vi "VI Snippets.vi"(6 "args":string[](array[string]), 7 "QD Plugins Dir":path, 8 "error in (no error)":errorcluster, 9 "Shift?":bool, 10 "Focus":enum8{"FP", "BD"}(ring), 11 "VI Refnum":refnum<vi>) -> (0 "error out":errorcluster)   [LabVIEW 2018]
doc: "Imports or exports a VI Snippet (*.png) image programmatically. Import opens a preview dialog to select a VI Snippet (*.png) from the <b>QuickDrop\\plugins\\Snippets</b> directory. Export prompts the user where to save the VI Snippet (*.png). On export, if nothing is selected the entire VI is exported. Otherwise only the selected Block Diagram GObjects are exported.\n\n[SCRIPT]\nimport=Import VI Snippet\nexport=Export VI Snippet"
uses:
  VI Snippets.llb/VI Snippets.lvlib
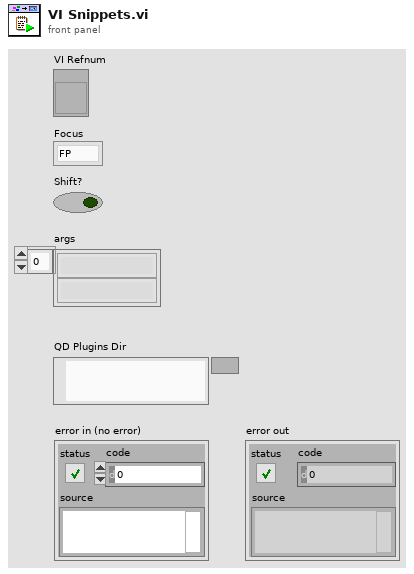
[diagram p1: front panel]
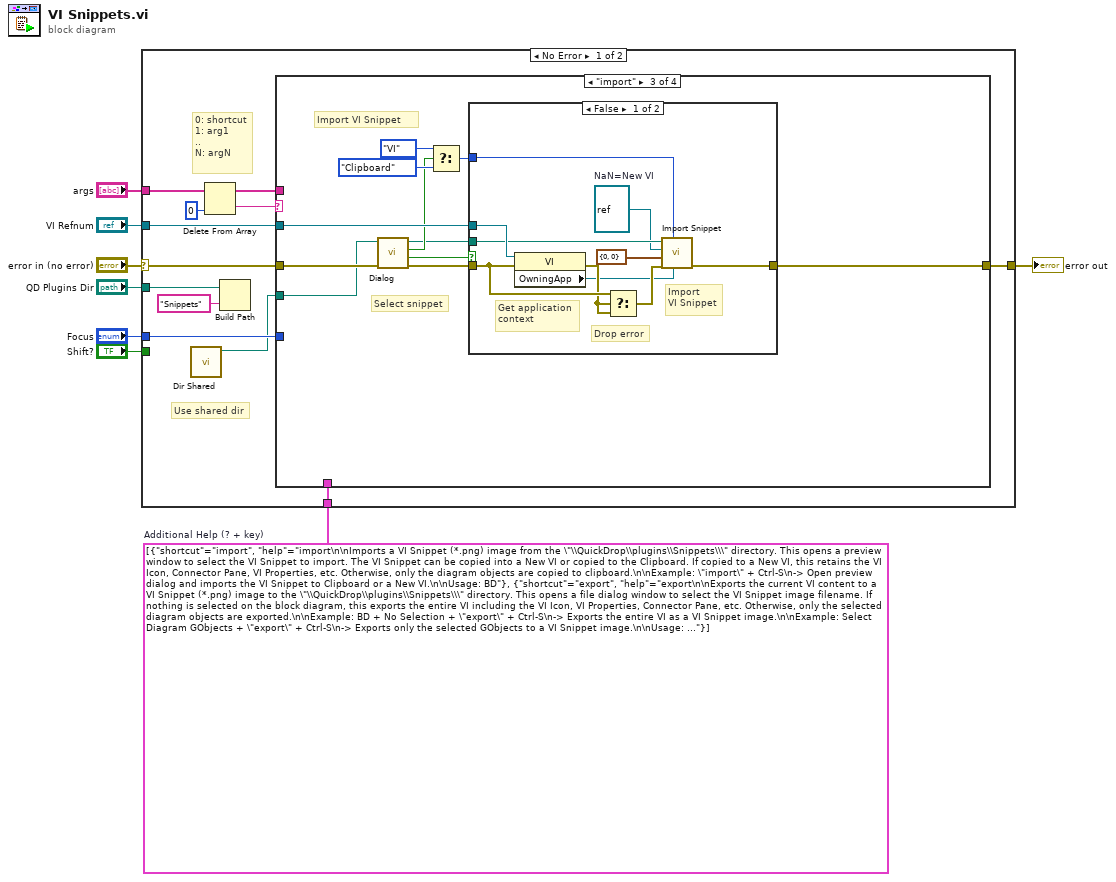
[diagram p0: block diagram]
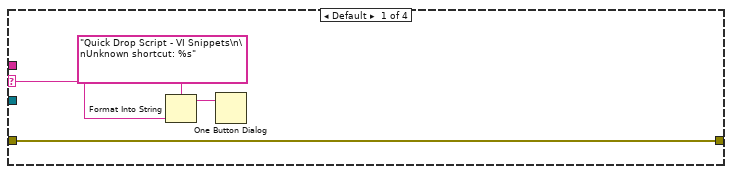
[diagram p2: hidden frame]
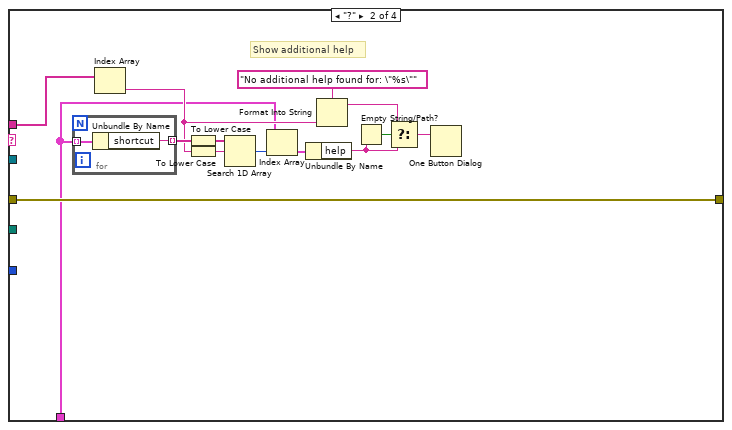
[diagram p3: hidden frame]
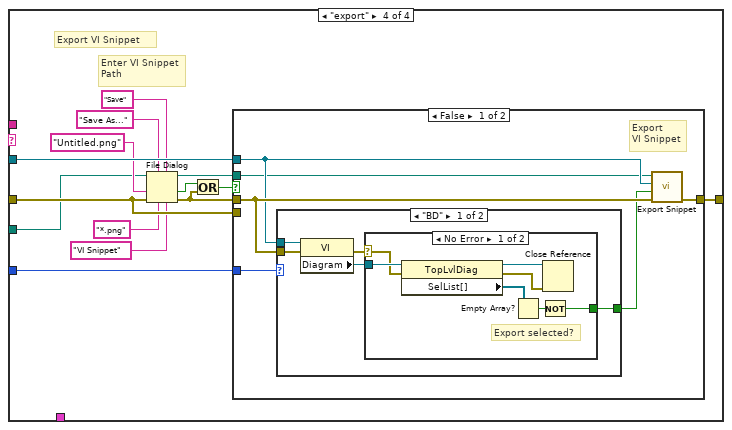
[diagram p5: hidden frame]
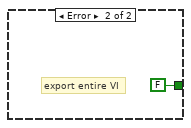
[diagram p6: hidden frame]
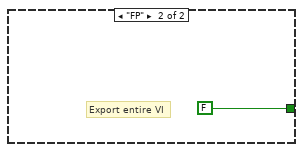
[diagram p7: hidden frame]
diagram:
  w1 = cluster{"shortcut":string, "help":string}[] [{"shortcut"="import", "help"="import\n\nImports a VI Snippet (*.png) image from the \"\\QuickDrop\\plugins\\Snippets\\\" directory. This opens a preview window to select the VI Snippet to import. The VI Snippet can be copied into a New VI or copied to the Clipboard. If copied to a New VI, this retains the VI Icon, Connector Pane, VI Properties, etc. Otherwise, only the diagram objects are copied to clipboard.\n\nExample: \"import\" + Ctrl-S\n-> Open preview dialog and imports the VI Snippet to Clipboard or a New VI.\n\nUsage: BD"}, {"shortcut"="export", "help"="export\n\nExports the current VI content to a VI Snippet (*.png) image to the \"\\QuickDrop\\plugins\\Snippets\\\" directory. This opens a file dialog window to select the VI Snippet image filename. If nothing is selected on the block diagram, this exports the entire VI including the VI Icon, VI Properties, Connector Pane, etc. Otherwise, only the selected diagram objects are exported.\n\nExample: BD + No Selection + \"export\" + Ctrl-S\n-> Exports the entire VI as a VI Snippet image.\n\nExample: Select Diagram GObjects + \"export\" + Ctrl-S\n-> Exports only the selected GObjects to a VI Snippet image.\n\nUsage: BD\n"}]  # Additional Help (? + key)
  n1 = case shown="No Error" "error in (no error)" {
    selector: "error in (no error)" -> [w16 w98]
    tunnel: "VI Refnum" -> [w12 _]
    tunnel: "Focus" -> [w11 _]
    tunnel: "Shift?" -> [_ _]
    tunnel: "args" -> [w19 _]
    tunnel: [w15 w98] -> w3
    tunnel: "QD Plugins Dir" -> [w14 _]
    tunnel: w1 -> [w10 _]
    frame No Error {
      # "Use shared dir"
      # "0: shortcut\n1: arg1\n..\nN: argN"
      n2 = call "Dir Shared.vi"() -> ("Shared Dir"=w9:path)  [unwired: 11 in]
      n3 = Delete From Array(array=w19, index=0) -> (deleted portion=w18:string, array with subset deleted=w17:string[])  [unwired: 1 in]
      n4 = Build Path(base path=w14, name or relative path="Snippets") -> ()  [unwired: 1 out]
      n5 = case shown="\"import\"" w18 {
        selector: w18 -> [w21 _ _ _]
        tunnel: [w24 w26 w51 w75] -> w15
        tunnel: w16 -> [w24 w26 w46 w72]
        tunnel: w17 -> [_ w27 _ _]
        tunnel: w9 -> [_ _ w42 w70]
        tunnel: w12 -> [_ _ w50 w74]
        tunnel: w11 -> [_ _ _ w73]
        tunnel: w10 -> [_ w25 _ _]
        frame Default {
          n6 = Format Into String(format string="Quick Drop Script - VI Snippets\n\nUnknown shortcut: %s", w21) -> (resulting string=w22:string)  [unwired: 2 in, 1 out]
          n7 = One Button Dialog(message=w22) -> ()  [unwired: 1 in, 1 out]
        }
        frame "?" {
          # "Show additional help"
          n8 = for {
            tunnel: w25 -> [w40] mode=indexing
            tunnel: [w39] -> w38 mode=indexing
            n9 = Unbundle By Name(w40) -> ("shortcut"=w39:string)
          }
          n10 = Index Array(array=w27) -> (element=w30:string)  [unwired: 1 in]
          n11 = To Lower Case(string=w38) -> (all lower case string=w37:string[])
          n12 = To Lower Case(string=w30) -> (all lower case string=w36:string)
          n13 = Search 1D Array(1D array=w37, element=w36) -> (index of element=w35:i32)  [unwired: 1 in]
          n14 = Index Array(array=w25, index=w35) -> (element=w34:cluster{"shortcut":string, "help":string})
          n15 = Unbundle By Name(w34) -> ("help"=w32:string)
          n16 = Format Into String(format string="No additional help found for: \"%s\"", w30) -> (resulting string=w29:string)  [unwired: 2 in, 1 out]
          n17 = Empty String/Path?(string/path=w32) -> (empty?=w33:bool)
          n18 = Select(t=w29, s=w33, f=w32) -> (s? t:f=w31:string)
          n19 = One Button Dialog(message=w31) -> ()  [unwired: 1 in, 1 out]
        }
        frame "import" {
          # "Import VI Snippet"
          # "Select snippet"
          n20 = call "Dialog.vi"("error in (no error)"=w46, "VI Snippets Dir"=w42) -> ("error out"=w45:errorcluster, "Cancelled?"=w44:bool, "New VI?"=w43:bool, "VI Snippets Path"=w41:path)  [unwired: 6 in]
          n21 = Select(t=enum8{"VI", "Clipboard"}."VI" ("Copy to (\"VI\")"), s=w43, f=enum8{"VI", "Clipboard"}."Clipboard" ("Copy to (\"VI\")")) -> (s? t:f=w47:enum8{"VI", "Clipboard"})
          n22 = case shown="False" w44 {
            tunnel: w45 -> [w60 w62]
            tunnel: [w56 w62] -> w51
            tunnel: w41 -> [w55 _]
            tunnel: w50 -> [w61 _]
            tunnel: w47 -> [w58 _]
            frame False {
              w54 = refnum<vi> refnum  # NaN=New VI
              # "Drop error"
              # "Get application\ncontext"
              # "Import\nVI Snippet"
              n23 = property class="VI"(reference=w61, error in=w60) -> (error out=w59:errorcluster, "OwningApp"=w52:refnum<vi>)  [unwired: 1 out]
              n24 = Select(t=w60, s=w59, f=w59) -> (s? t:f=w57:errorcluster)
              n25 = call "Import Snippet.vi"("App Refnum (New VI only)"=w52, "Copy to (\"VI\")"=w58, "error in (no error)"=w57, "Drop Position (0, 0)"=cluster{"Left":i32, "Top":i32} {"Left"=0, "Top"=0}, "VI Refnum in (NaN=New VI)"=w54, "VI Snippet Path (*.png)"=w55) -> ("error out"=w56:errorcluster)  [unwired: 2 in, 3 out]
            }
            frame True {
              # "Cancelled"
            }
          }
        }
        frame "export" {
          # "Export VI Snippet"
          # "Enter VI Snippet\nPath"
          n26 = File Dialog(4:"VI Snippet" ("pattern label"), 5:"Save" ("button label"), 6:"*.png" ("pattern (all files)"), 7:"Save As..." ("prompt"), 8:w72, 9:"Untitled.png" ("default name"), 11:w70) -> (0:w69:errorcluster, 1:w68:bool, 3:w67:path)  [unwired: 1 out]
          n27 = Or(x=w68, y=w69) -> (x .or. y?=w76:bool)
          n28 = case shown="False" w76 {
            tunnel: w72 -> [_ w97]
            tunnel: [w77 w97] -> w75
            tunnel: w67 -> [w78 _]
            tunnel: w69 -> [w81 _]
            tunnel: w74 -> [w79 _]
            tunnel: w73 -> [w82 _]
            frame False {
              # "Export\nVI Snippet"
              n29 = case shown="\"BD\"" w82 {
                tunnel: [w84 FALSE ("Selected GObjects Only? (F)")] -> w80
                tunnel: w79 -> [w87 _]
                tunnel: w81 -> [w83 _]
                frame "BD" {
                  n30 = property class="VI"(reference=w87, error in=w83) -> (error out=w85:errorcluster, "Diagram"=w86:refnum<vi>)  [unwired: 1 out]
                  n31 = case shown="No Error" w85 {
                    selector: w85 -> [w93 _]
                    tunnel: w86 -> [w94 _]
                    tunnel: [w88 FALSE] -> w84
                    frame No Error {
                      # "Export selected?"
                      n32 = property class="TopLvlDiag"(reference=w94, error in=w93) -> (reference out=w91:refnum<vi>, error out=w90:errorcluster, "SelList[]"=w92:refnum<vi>[])
                      n33 = Empty Array?(array=w92) -> (empty?=w89:bool)
                      n34 = Not(x=w89) -> (.not. x?=w88:bool)
                      n35 = Close Reference(reference=w91, error in (no error)=w90) -> ()  [unwired: 1 out]
                    }
                    frame Error {
                      # "export entire VI"
                    }
                  }
                }
                frame "FP" {
                  # "Export entire VI"
                }
              }
              n36 = call "Export Snippet.vi"("error in (no error)"=w81, "Selected GObjects Only? (F)"=w80, "VI Refnum"=w79, "VI Snippet Path (*.png)"=w78) -> ("error out"=w77:errorcluster)  [unwired: 5 in, 2 out]
            }
            frame True {
              # "Cancelled"
            }
          }
        }
      }
    }
    frame Error {
    }
  }
  "error out" <- w3
